vi "TimedTrigger.vi"(8 "error in (no error)":errorcluster, 10 "clTimedTrigger":T1={"TriggerName"="", "Time after next UTC Second"=0.0, "Trigger Duration"=0.1}, 11 "PXI_MultiTrig in":refnum<class "PXI_MultiTrig.lvclass">) -> (0 "error out":errorcluster, 3 "PXI_MultiTrig out":refnum<class "PXI_MultiTrig.lvclass">)   [LabVIEW 2018, in "SyncPlugins.lvlib" / "PXI_MultiTrig.lvclass"]
uses:
  PXI_MultiTrig.lvclass
  SyncPluginBase/Typedefs/clTimedTrigger.ctl
  PXI_MultiTrig.lvclass/PXI_MultiTrig.ctl
  Accessors/Read RefClkSession.vi
  Accessors/Write RefClkSession.vi
  Accessors/Write Triggers.vi
  Accessors/Read Triggers.vi
  <vilib>/Utility/error.llb/Error Cluster From Error Code.vi
  <vilib>/ErrorRing/Error Ring.xnode
  SyncPluginBase/SyncPluginBase.lvclass
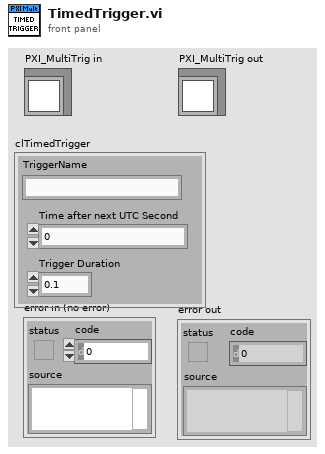
[diagram p1: front panel]
types:
  T1 = typedef "SyncPlugins.lvlib/SyncPluginBase.lvclass/clTimedTrigger.ctl" = cluster{"TriggerName":string, "Time after next UTC Second":dbl, "Trigger Duration":dbl}
  T2 = typedef "SyncPlugins.lvlib/PXI_MultiTrig.lvclass/clTrigger.ctl" = cluster{"Name":string, "DestTerm":string, "SrcTerm":string, "SyncClk":string, "Edge":i32, "Invert?":i32, "Initiated":bool, "Type":string, "TrigTime":bool}
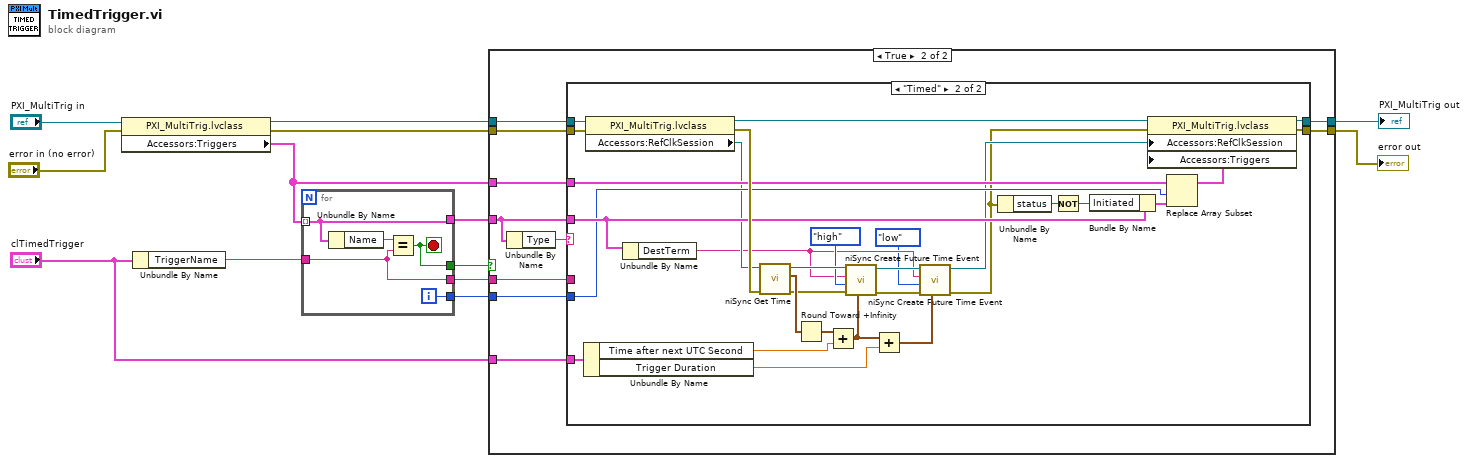
[diagram p0: block diagram]
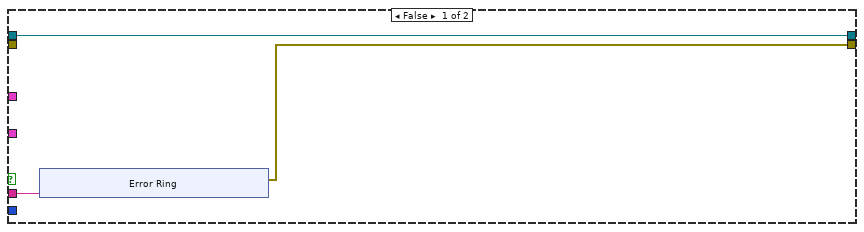
[diagram p2: hidden frame]
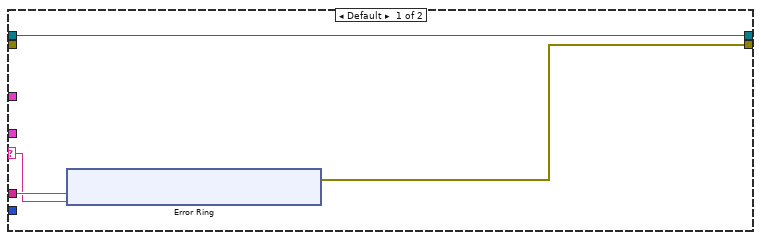
[diagram p3: hidden frame]
diagram:
  n1 = property class="PXI_MultiTrig.lvclass"(reference="PXI_MultiTrig in", error in="error in (no error)") -> (reference out=w8:refnum<class "PXI_MultiTrig.lvclass">, error out=w7:errorcluster, "Accessors:Triggers"=w2:T2[])
  n2 = Unbundle By Name("clTimedTrigger") -> ("TriggerName"=w11:string)
  n3 = for {
    tunnel: w2 -> [w17] mode=indexing
    tunnel: w11 -> [w15]
    tunnel: [w17] -> w4
    tunnel: [w16] -> w10
    tunnel: [w15] -> w9
    tunnel: [w14] -> w3
    i -> [w14]
    stop <- w16 stop-if-true
    n4 = Unbundle By Name(w17) -> ("Name"=w18:string)
    n5 = Equal?(x=w18, y=w15) -> (x = y?=w16:bool)
  }
  n6 = case shown="True" w10 {
    tunnel: w9 -> [w21 w37]
    tunnel: w8 -> [w20 w32]
    tunnel: w7 -> [_ w30]
    tunnel: [w20 w31] -> w6
    tunnel: [w19 w34] -> w5
    tunnel: w4 -> [_ w33]
    tunnel: w3 -> [_ w36]
    tunnel: w2 -> [_ w35]
    tunnel: "clTimedTrigger" -> [_ w29]
    frame False {
      n7 = xnode "Error Ring"("parameter 0"=w21) -> ("error out"=w19:errorcluster)
    }
    frame True {
      n8 = Unbundle By Name(w33) -> ("Type"=w38:string)
      n9 = case shown="\"Timed\"" w38 {
        selector: w38 -> [w41 _]
        tunnel: w37 -> [w42 _]
        tunnel: w36 -> [_ w66]
        tunnel: w35 -> [_ w67]
        tunnel: [w40 w72] -> w34
        tunnel: w33 -> [_ w71]
        tunnel: w32 -> [w39 w79]
        tunnel: [w39 w73] -> w31
        tunnel: w30 -> [_ w80]
        tunnel: w29 -> [_ w53]
        frame Default {
          n10 = xnode "Error Ring"("parameter 0"=w42, "parameter 1"=w41) -> ("error out"=w40:errorcluster)
        }
        frame "Timed" {
          n11 = Unbundle By Name(w53) -> ("Time after next UTC Second"=w52:dbl, "Trigger Duration"=w51:dbl)
          n12 = property class="PXI_MultiTrig.lvclass"(reference=w79, error in=w80) -> (reference out=w74:refnum<class "PXI_MultiTrig.lvclass">, error out=w78:errorcluster, "Accessors:RefClkSession"=w64:refnum<k15>)
          n13 = Unbundle By Name(w71) -> ("DestTerm"=w57:string)
          n14 = call <instrlib>:"niSync Get Time.vi"("error in (no error)"=w78, "instrument handle"=w64) -> ("error out"=w75:errorcluster, "time"=w77:timestamp, "instrument handle out"=w63:refnum<k15>)  [unwired: 5 in]
          n15 = Round Toward +Infinity(x=w77) -> (ceil(x): smallest int >= x=w76:timestamp)
          n16 = Add(x=w76, y=w52) -> (x+y=w59:timestamp)
          n17 = call <instrlib>:"niSync Create Future Time Event.vi"("time"=w59, "error in (no error)"=w75, "output level"=enum32{"low", "high"}."high", "terminal"=w57, "instrument handle"=w63) -> ("error out"=w61:errorcluster, "instrument handle out"=w60:refnum<k15>)  [unwired: 4 in]
          n18 = Add(x=w59, y=w51) -> (x+y=w58:timestamp)
          n19 = call <instrlib>:"niSync Create Future Time Event.vi"("time"=w58, "error in (no error)"=w61, "output level"=enum32{"low", "high"}."low", "terminal"=w57, "instrument handle"=w60) -> ("error out"=w54:errorcluster, "instrument handle out"=w55:refnum<k15>)  [unwired: 4 in]
          n20 = Unbundle By Name(w54) -> ("status"=w70:bool)
          n21 = Not(x=w70) -> (.not. x?=w69:bool)
          n22 = Bundle By Name(cluster=w71, "Initiated"=w69) -> (w68:T2)
          n23 = Replace Array Subset(array=w67, new element=w68, index=w66) -> (w65:T2[])
          n24 = property class="PXI_MultiTrig.lvclass"(reference=w74, error in=w54, "Accessors:RefClkSession"=w55, "Accessors:Triggers"=w65) -> (reference out=w73:refnum<class "PXI_MultiTrig.lvclass">, error out=w72:errorcluster)
        }
      }
    }
  }
  "error out" <- w5
  "PXI_MultiTrig out" <- w6
